vi "Get State.vi"(8 "error in (no error)":errorcluster, 11 "Red Pitaya Digitizer in":refnum<class "Red Pitaya Digitizer.lvclass">) -> (0 "error out":errorcluster, 1 "Data ready":bool, 2 "Armed":bool, 3 "Red Pitaya Digitizer out":refnum<class "Red Pitaya Digitizer.lvclass">, 4 "Availiable Samples":u32, 5 "Finished":bool)   [LabVIEW 2016, in "Red Pitaya Digitizer.lvclass"]
uses:
  Red Pitaya Digitizer.lvclass
  Red Pitaya Digitizer.lvclass/Red Pitaya Digitizer.ctl
  Read RP Instrument.vi
  Write RP Instrument.vi
  RP Core/RP Instrument/RP Instrument.lvclass
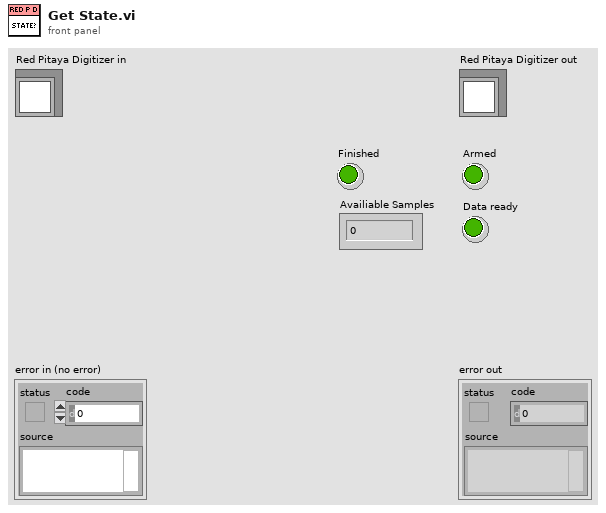
[diagram p1: front panel]
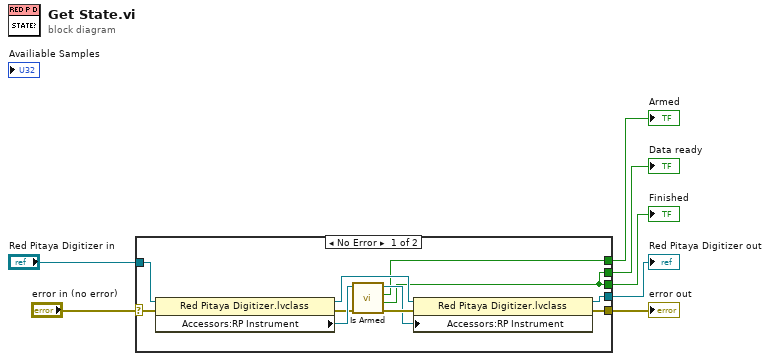
[diagram p0: block diagram]
diagram:
  n1 = case shown="No Error" "error in (no error)" {
    selector: "error in (no error)" -> [w15 w20]
    tunnel: "Red Pitaya Digitizer in" -> [w18 w19]
    tunnel: [w11 w19] -> w5
    tunnel: [w10 w20] -> w4
    tunnel: [w9 _] -> w3
    tunnel: [w8 _] -> w2
    tunnel: [w8 _] -> w1
    frame No Error {
      n2 = property class="Red Pitaya Digitizer.lvclass"(reference=w18, error in=w15) -> (reference out=w14:refnum<class "Red Pitaya Digitizer.lvclass">, error out=w16:errorcluster, "Accessors:RP Instrument"=w17:refnum<class "RP Instrument.lvclass">)
      n3 = call-dynamic "Is Armed.vi"("error in (no error)"=w16, "RP Instrument in"=w17) -> ("error out"=w13:errorcluster, "Finished"=w8:bool, "Armed"=w9:bool, "RP Instrument out"=w12:refnum<class "RP Instrument.lvclass">)  [unwired: 6 in]
      n4 = property class="Red Pitaya Digitizer.lvclass"(reference=w14, error in=w13, "Accessors:RP Instrument"=w12) -> (reference out=w11:refnum<class "Red Pitaya Digitizer.lvclass">, error out=w10:errorcluster)
    }
    frame Error {
    }
  }
  "error out" <- w4
  "Red Pitaya Digitizer out" <- w5
  "Armed" <- w3
  "Data ready" <- w2
  "Finished" <- w1
